vi "Safety Config Arcade Drive.vi"() -> ()   [LabVIEW 2025]
doc: "Safety Config Arcade Drive example\n\nThis example shows how Safety Config is used for RobotDrive outputs. By default Safety Config is enabled for RobotDrive. This means that RobotDrive must be called at least every 100 ms. Otherwise the motor outputs will be turned off until RobotDrive gets called.\n\n1. Set up your robot and wiring.\n2. Run this VI.\n3. Increase the loop delay to 300 ms. This simulates what happens if other code is starving the drive loop code. When the loop delay is large enough, the Safety Config will turn off the RobotDrive motors. You will likely see the motors pulse on and off, because when Safety Config is enabled RobotDrive needs to be called at least every 100 ms.\n4. With the loop delay still at 300 ms, Select <B>Safety Config Off</B>. This disables Safety Config - you can disable as needed in your program.\n\nThis example uses radio buttons to enable and disable Safety Config.\n\nThis example expects a USB cable connected from your development PC to the Type B USB Jack (next to the power input) on the roboRIO.\n\nThis example requires the Driver Station to be running with Teleoperated Enabled."
uses:
  <vilib>/Rock Robotics/SystemInterfaces/DIO/FPGA_DIOPWMChannel.ctl
  <vilib>/Rock Robotics/WPI/Joystick/WPI_JoystickDeviceEnum.ctl
  <vilib>/Rock Robotics/WPI/SafetyOutput/WPI_SafetyOutputConfigMenu.ctl
  <vilib>/Rock Robotics/WPI/RobotDrive/WPI_RobotDriveOpen2MotorWithTalon.vi
  <vilib>/Rock Robotics/WPI/RobotDrive/WPI_RobotDriveArcadeDrive_Standard(NoSaturation).vi
panel:
  in  "safety config":enum32{"Safety Config On ", "Safety Config Off"}(radio)
  in  "loop delay (ms)":u32(slide) scale=0.0..300.0
  in  "Joystick":T1
  in  "Left Motor (PWM channel)":T2
  in  "Right Motor (PWM channel)":T2=enum."PWM 1"
  in  "stop":bool
  # "Set these inputs before running."
  # "These can be set while running."
  # "This example requires the Driver Station to be running with Teleoperated Enabled."
  # "PWM cables"
  # "This shows wiring for Talon speed controllers.  The wiring is similar for other motor controllers.  If you change the controller type, you must also select the appropriate instance of the Motor Open VI on the diagram."
  # "Power\nTerminals"
  # "Motor\nTerminals"
  # "+"
  # "+"
  # "M"
  # "B"
  # "Power\nTerminals"
  # "Motor\nTerminals"
  # "+"
  # "+"
  # "M"
  # "B"
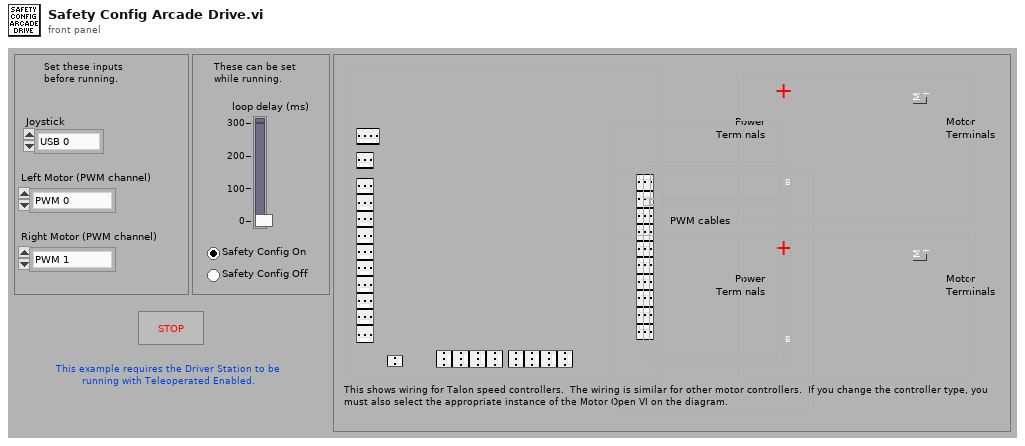
[diagram p1: front panel]
types:
  T1 = typedef "WPI_JoystickDeviceEnum.ctl" = enum16{"USB 0", "USB 1", "USB 2", "USB 3", "USB 4", "USB 5"}
  T2 = typedef "FPGA_DIOPWMChannel.ctl" = enum8{"PWM 0", "PWM 1", "PWM 2", "PWM 3", "PWM 4", "PWM 5", "PWM 6", "PWM 7", "PWM 8", "PWM 9", "PWM MXP 0", "PWM MXP 1", "PWM MXP 2", "PWM MXP 3", "PWM MXP 4", "PWM MXP 5", "PWM MXP 6", "PWM MXP 7", "PWM MXP 8", "PWM MXP 9", "Invalid"}
  T3 = typedef "WPI_JoystickDevRef.ctl" = cluster{"Device":T1}
  T4 = typedef "WPI_RobotDriveDevRef.ctl" = cluster{"DevStatus":errorcluster, "Motors[]":T5[], "Square Inputs":bool, "Max Output":dbl}
  T5 = typedef "WPI_MotorControlDeviceRef.ctl" = cluster{"DeviceStatus":errorcluster, "Type":T6, "PWM":cluster{"PWM Channel":T2, "DeadBand":T7}, "CAN":cluster{"Device Number":u8, "SetOutput VI Ref":variant, "GetOutput VI Ref":variant, "Enable VI Ref":variant, "Disable VI Ref":variant, "Data":variant}, "Invert":bool, "DIO PWM":cluster{"PWM \"Enable\" Channel":T2, "DIOChannel":T8, "PWM Rate":dbl}}
  T6 = typedef "WPI_MotorControlType.ctl" = enum16{"PWM", "CAN", "DIO PWM"}
  T7 = typedef "WPI_PWMDeadband.ctl" = cluster{"Name":string, "maxPositivePwm":i32, "minPositivePwm":i32, "centerPwm":i32, "maxNegativePwm":i32, "minNegativePwm":i32, "angularRange":u16}
  T8 = typedef "FPGA_DIOChannel.ctl" = enum8{"DIO 0", "DIO 1", "DIO 2", "DIO 3", "DIO 4", "DIO 5", "DIO 6", "DIO 7", "DIO 8", "DIO 9", "DIO MXP 0", "DIO MXP 1", "DIO MXP 2", "DIO MXP 3", "DIO MXP 4", "DIO MXP 5", "DIO MXP 6", "DIO MXP 7", "DIO MXP 8", "DIO MXP 9", "DIO MXP 10", "DIO MXP 11", "DIO MXP 12", "DIO MXP 13", "DIO MXP 14", "DIO MXP 15", "SPI Port CS1", "SPI Port CS2", "SPI Port CS3", "SPI Port MISO", "SPI Port MOSI", "Invalid"}
  T9 = typedef "WPI_SafetyOutputConfigMenu.ctl" = enum16{"Enable", "Disable"}
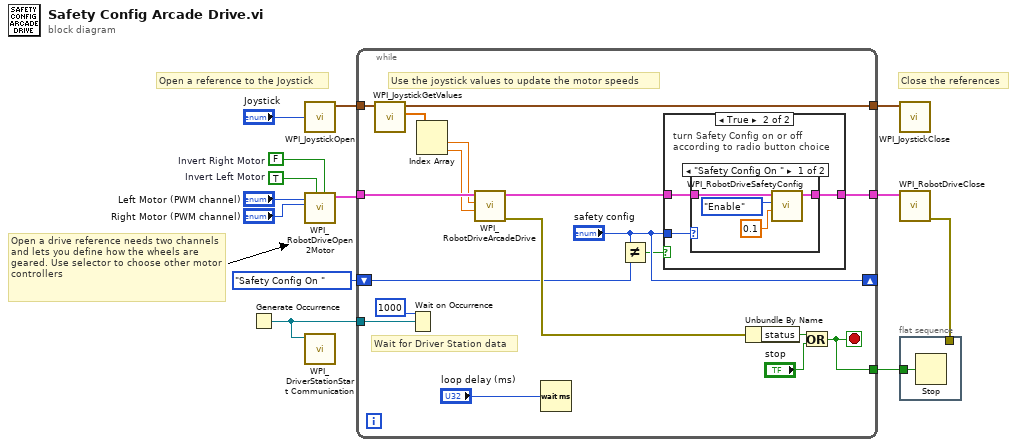
[diagram p0: block diagram]
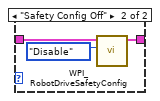
[diagram p3: hidden frame]
diagram:
  w7 = FALSE  # Invert Right Motor
  w8 = TRUE  # Invert Left Motor
  # "Open a reference to the Joystick"
  # "Close the references"
  # "Open a drive reference needs two channels and lets you define how the wheels are geared. Use selector to choose other motor controllers"
  n1 = Generate Occurrence() -> (w9:refnum<k4>)
  n2 = call <vilib>:"WPI_JoystickOpen.vi"("JoystickDevice"="Joystick") -> ("JoystickDevRef"=w5:T3)  [unwired: 10 out]
  n3 = call-poly <vilib>:"WPI_RobotDriveOpen2Motor.vi"("Right Motor Inverted"=w7, "Left Motor Inverted"=w8, "Right Motor"="Right Motor (PWM channel)", "Left Motor"="Left Motor (PWM channel)") -> ("RobotDriveDevRef"=w11:T4)  [unwired: 1 in, 6 out]
  n4 = call <vilib>:"WPI_DriverStationStart Communication.vi"("occurrence"=w9) -> ()  [unwired: 2 in, 9 out]
  n5 = while {
    tunnel: w11 -> [w28]
    tunnel: [w20] -> w10
    tunnel: [w24] -> w2
    tunnel: w9 -> [w31]
    tunnel: w5 -> [w29]
    tunnel: [w16] -> w4
    shift-right: ["safety config"] -> _
    shift-left: enum32{"Safety Config On ", "Safety Config Off"}."Safety Config On " ("safety config") -> [w19]
    stop <- w24 stop-if-true
    # "Wait for Driver Station data"
    # "Use the joystick values to update the motor speeds"
    n6 = call <vilib>:"WPI_JoystickGetValues.vi"("JoystickDevRef"=w29) -> ("Axes"=w23:dbl[], "JoystickDevRef"=w16:T3)  [unwired: 6 in, 3 out]
    n7 = Wait on Occurrence(2:w31, 3:1000 ("ms timeout (-1)")) -> ()  [unwired: 2 out]
    n8 = Index Array(array=w23) -> (element #1=w15:dbl, element #2=w14:dbl)  [unwired: 2 in]
    n9 = call-poly <vilib>:"WPI_RobotDriveArcadeDrive.vi"("Y axis value"=w14, "X axis value"=w15, "RobotDriveDevRef"=w28) -> ("error out"=w27:errorcluster, "RobotDriveDevRef"=w21:T4)  [unwired: 1 in, 6 out]
    n10 = Wait (ms)(milliseconds to wait="loop delay (ms)") -> ()  [unwired: 1 out]
    n11 = Not Equal?(x="safety config", y=w19) -> (x != y?=w17:bool)
    n12 = case shown="True" w17 {
      tunnel: w21 -> [w32 w35]
      tunnel: [w32 w34] -> w20
      tunnel: "safety config" -> [_ w33]
      frame False {
        # "don't change Safety Config"
      }
      frame True {
        # "turn Safety Config on or off according to radio button choice"
        n13 = case shown="\"Safety Config On \"" w33 {
          tunnel: w35 -> [w39 w41]
          tunnel: [w38 w40] -> w34
          frame "Safety Config On " {
            n14 = call <vilib>:"WPI_RobotDriveSafetyConfig.vi"("timeout (s)"=0.1, "mode"=WPI_SafetyOutputConfigMenu."Enable", "RobotDriveDevRef"=w39) -> ("RobotDriveDevRef"=w38:T4)  [unwired: 1 in, 7 out]
          }
          frame "Safety Config Off" {
            n15 = call <vilib>:"WPI_RobotDriveSafetyConfig.vi"("mode"=WPI_SafetyOutputConfigMenu."Disable", "RobotDriveDevRef"=w41) -> ("RobotDriveDevRef"=w40:T4)  [unwired: 2 in, 7 out]
          }
        }
      }
    }
    n16 = Unbundle By Name(w27) -> ("status"=w26:bool)
    n17 = Or(x=w26, y="stop") -> (x .or. y?=w24:bool)
  }
  n18 = call <vilib>:"WPI_JoystickClose.vi"("JoystickDevRef"=w4) -> ()  [unwired: 11 out]
  n19 = call <vilib>:"WPI_RobotDriveClose.vi"("RobotDriveDevRef"=w10) -> ("error out"=w1:errorcluster)  [unwired: 1 in, 9 out]
  n20 = flat-sequence {
    tunnel: w2 -> [w43]
    tunnel: w1 -> [_]
    frame #0 {
      n21 = Stop(stop? (T)=w43) -> ()
    }
  }
